vi "SV_Correction.vi"(8 "error in (no error)":errorcluster, 11 "Input Cluster":T3) -> (0 "error IO":errorcluster, 2 "Points for Array Overlay Out":T1(array[cluster]), 3 "Measurement Results":dbl[](array[numeric]))   [LabVIEW 2019, in "Algorithm.lvclass"]
uses:
  FrameworkOverrides/Algorithm.lvclass
  <vilib>/vision/NI_Vision_Development_Module.lvlib
  <vilib>/vision/Image Controls.llb/IMAQ Image.ctl
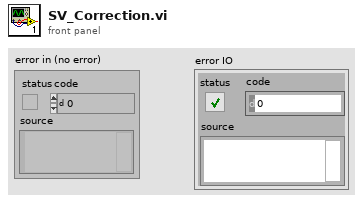
[diagram p1: front panel]
types:
  T1 = cluster{"Points for Arrow Overlay[0]":cluster{"X":sgl, "Y":sgl}, "Points for Arrow Overlay[1]":cluster{"X":sgl, "Y":sgl}, "Points for Arrow Overlay[2]":cluster{"X":sgl, "Y":sgl}, "Points for Arrow Overlay[3]":cluster{"X":sgl, "Y":sgl}}[]
  T2 = typedef "IMAQ Image.ctl" = refnum<image>
  T3 = cluster{"Side Calibration Image":T2, "Part Name":string, "Measurement Names Array":string[], "Measurement Results":dbl[], "Points for Array Overlay in":cluster{"Points for Arrow Overlay[0]":cluster{"X":sgl, "Y":sgl}, "Points for Arrow Overlay[1]":cluster{"X":sgl, "Y":sgl}, "Points for Arrow Overlay[2]":cluster{"X":sgl, "Y":sgl}, "Points for Arrow Overlay[3]":cluster{"X":sgl, "Y":sgl}}[]}
  T4 = cluster{"Points for Arrow Overlay[0]":cluster{"X":sgl, "Y":sgl}, "Points for Arrow Overlay[1]":cluster{"X":sgl, "Y":sgl}, "Points for Arrow Overlay[2]":cluster{"X":sgl, "Y":sgl}, "Points for Arrow Overlay[3]":cluster{"X":sgl, "Y":sgl}}
  T5 = cluster{"Pixel Coordinates":cluster{"X":sgl, "Y":sgl}, "Pixel Coordinates":cluster{"X":sgl, "Y":sgl}, "Points for Arrow Overlay[2]":cluster{"X":sgl, "Y":sgl}, "Points for Arrow Overlay[3]":cluster{"X":sgl, "Y":sgl}}
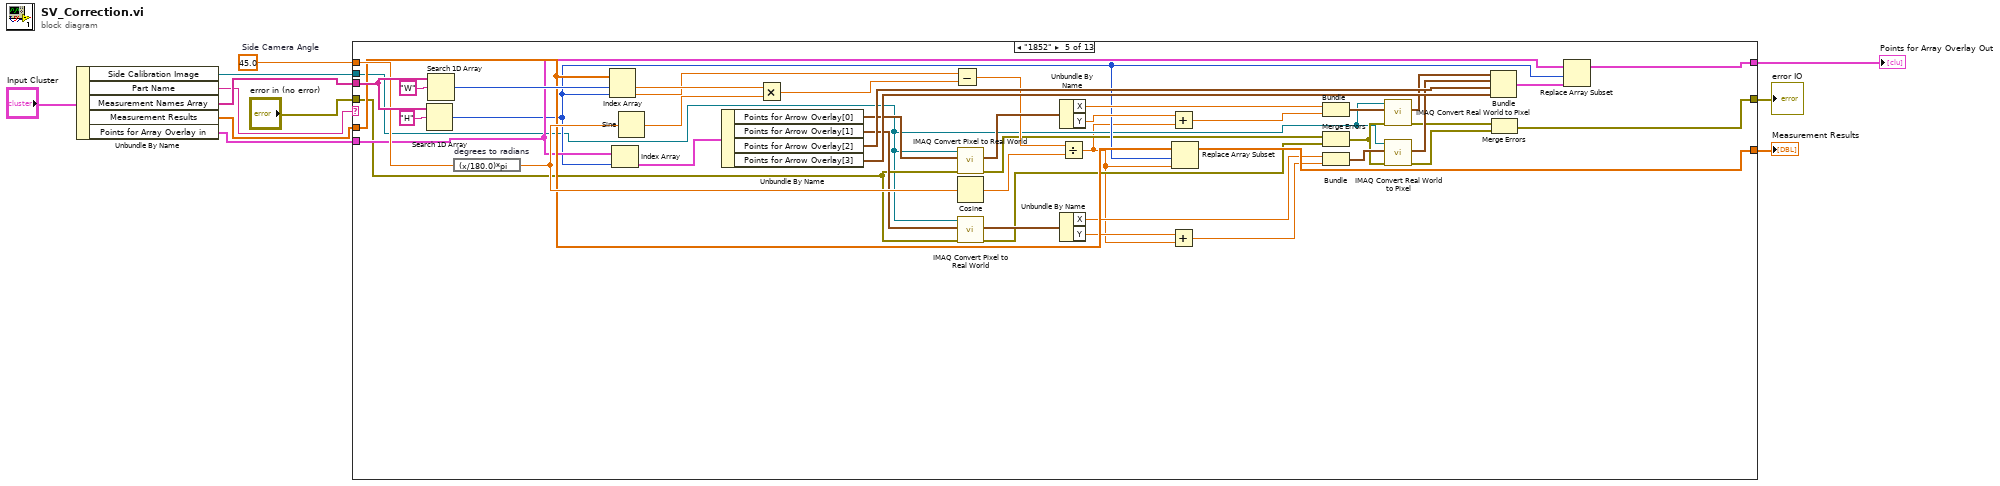
[diagram p0: block diagram]
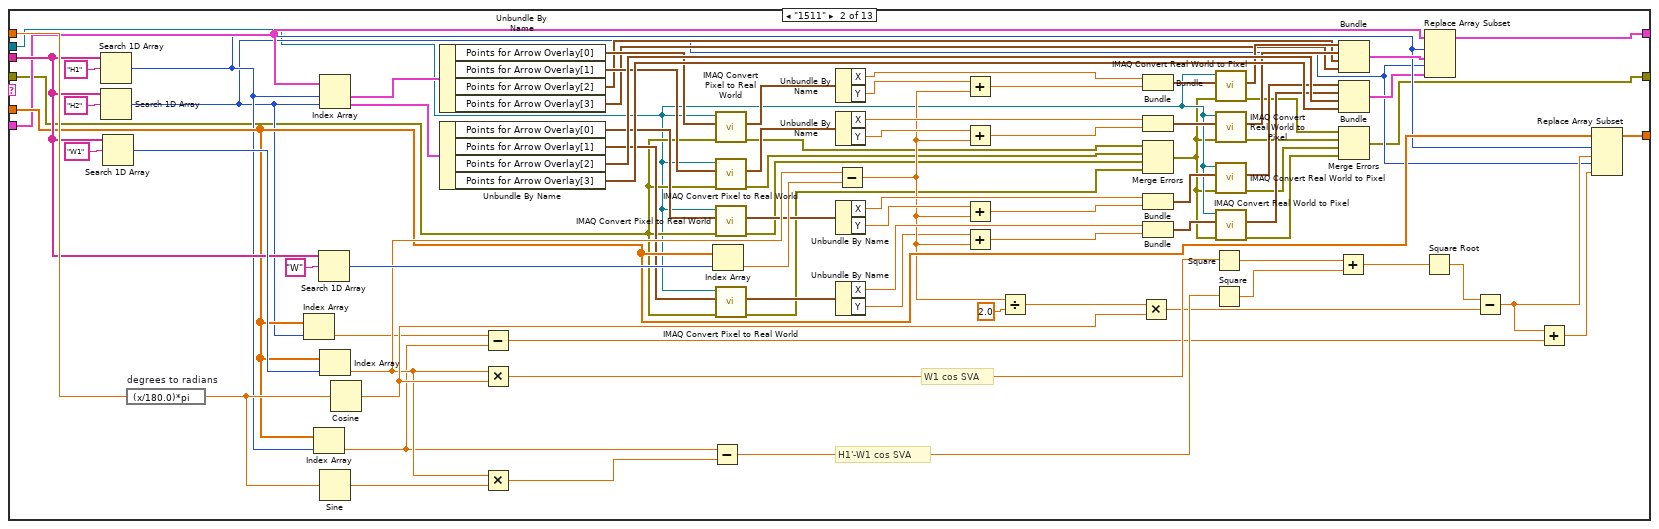
[diagram p3: hidden frame]
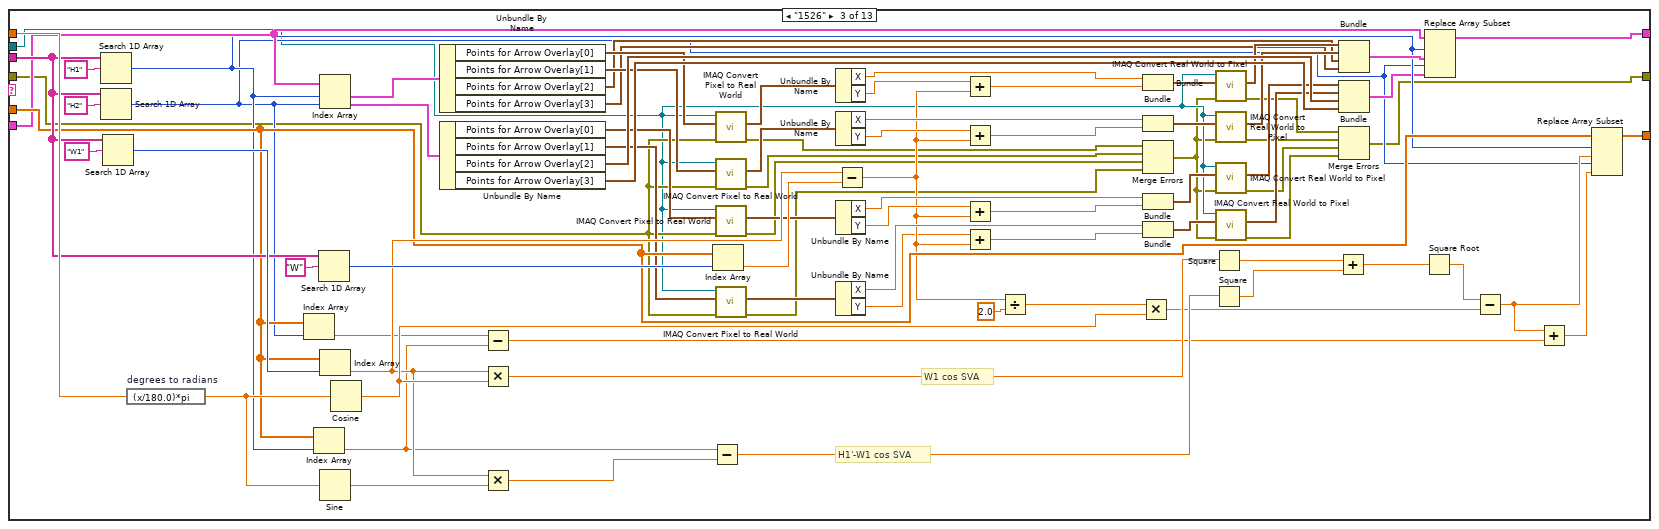
[diagram p4: hidden frame]
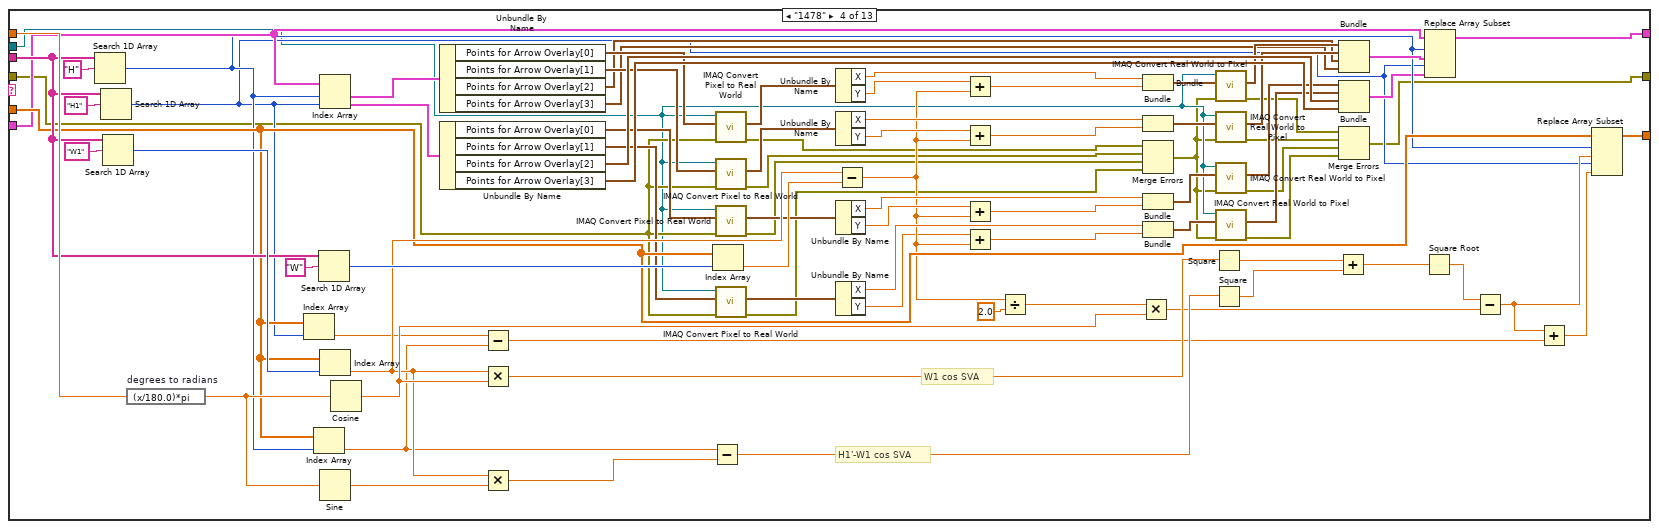
[diagram p5: hidden frame]
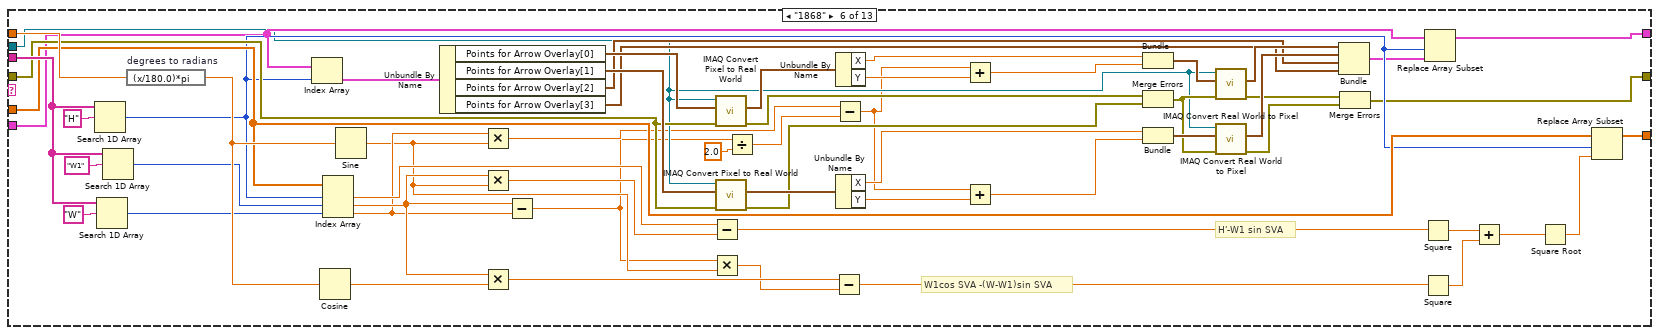
[diagram p6: hidden frame]
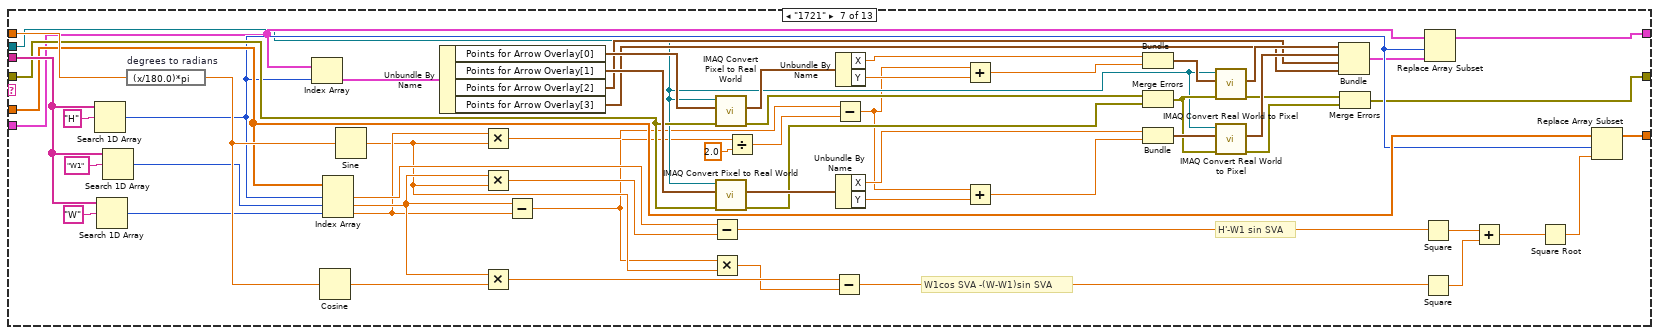
[diagram p7: hidden frame]
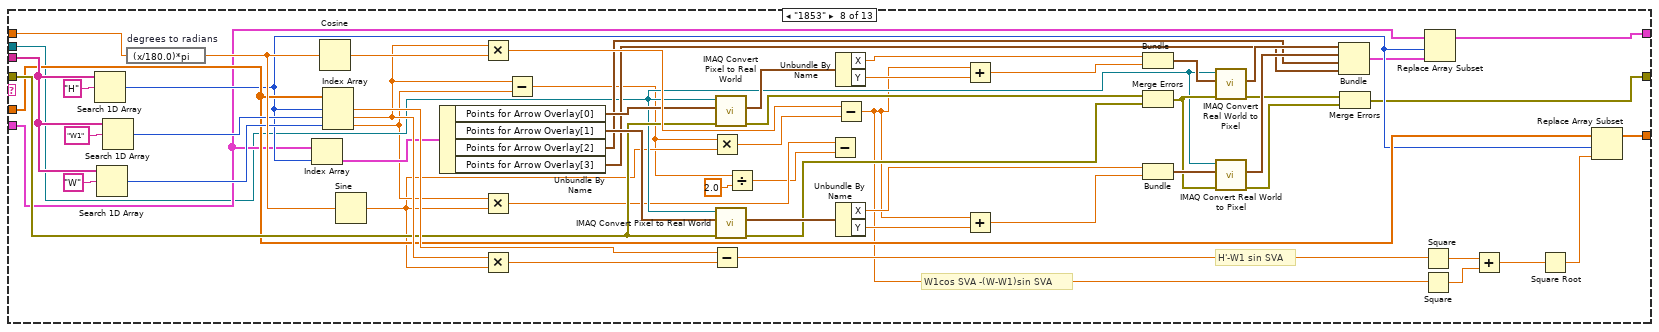
[diagram p8: hidden frame]
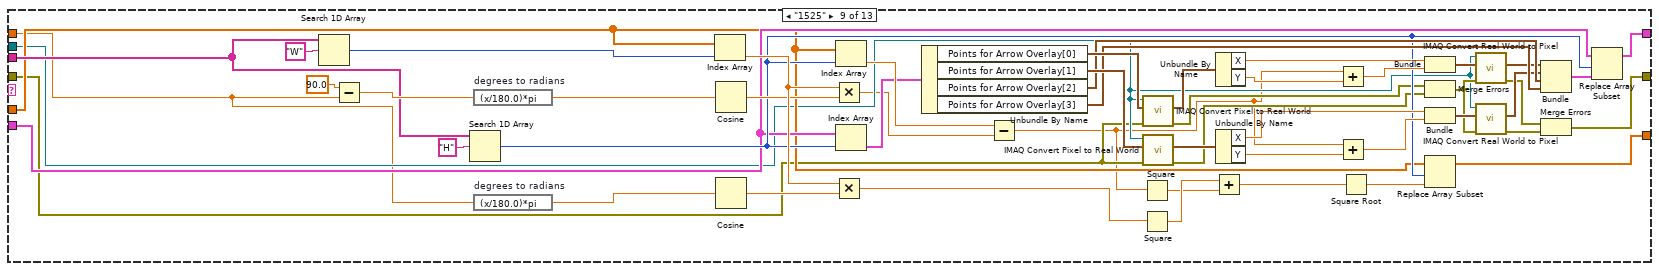
[diagram p9: hidden frame]
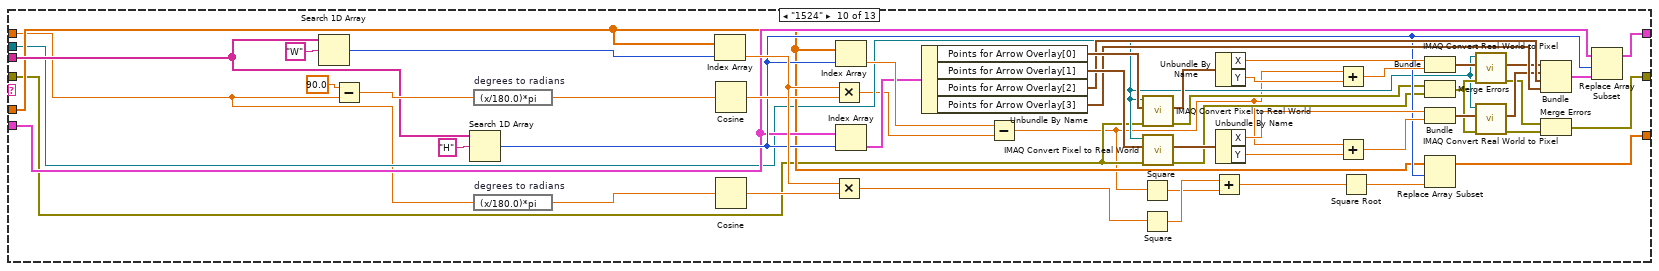
[diagram p10: hidden frame]
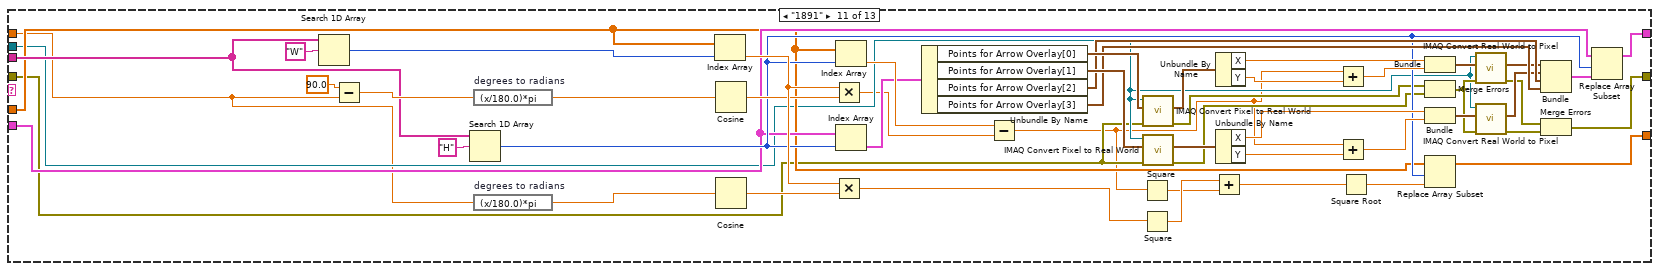
[diagram p11: hidden frame]
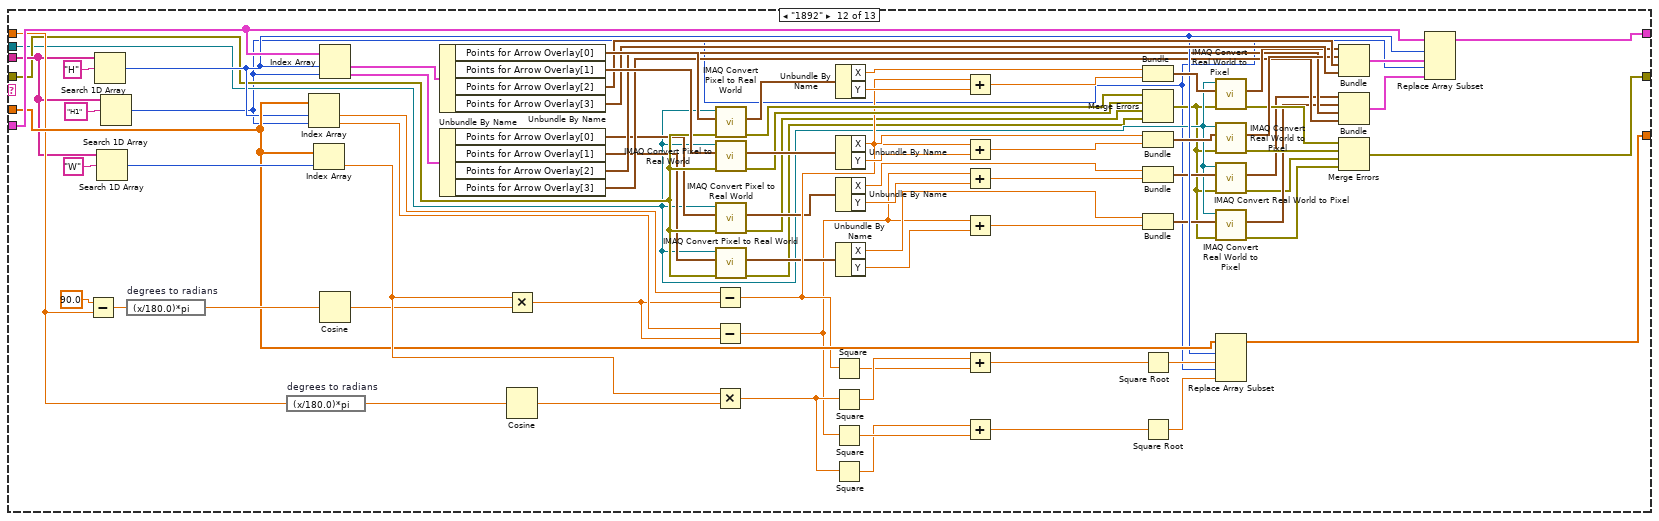
[diagram p12: hidden frame]
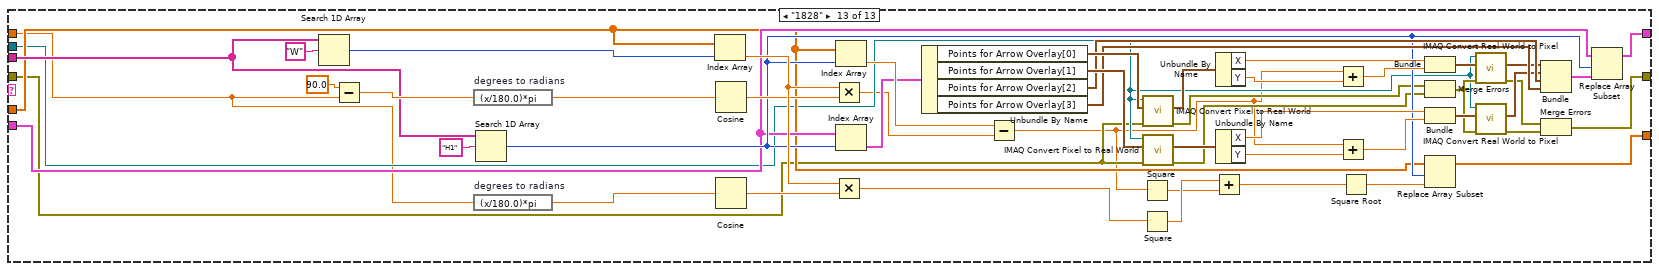
[diagram p13: hidden frame]
diagram:
  w10 = 45.0  # Side Camera Angle
  n1 = Unbundle By Name("Input Cluster") -> ("Side Calibration Image"=w5:T2, "Part Name"=w8:string, "Measurement Names Array"=w9:string[], "Measurement Results"=w7:dbl[], "Points for Array Overlay in"=w4:T1)
  n2 = case shown="\"1852\"" w8 {
    tunnel: w10 -> [_ w83 w166 w249 w299 w347 w405 w463 w487 w538 w589 w675 w721]
    tunnel: w9 -> [_ w78 w161 w244 w303 w355 w413 w471 w491 w542 w593 w669 w725]
    tunnel: w7 -> [w13 w71 w154 w237 w295 w325 w383 w441 w489 w540 w591 w676 w723]
    tunnel: [w13 w69 w152 w235 w294 w324 w382 w440 w485 w536 w587 w674 w719] -> w6
    tunnel: w5 -> [_ w20 w103 w186 w265 w316 w374 w432 w488 w539 w590 w643 w722]
    tunnel: w4 -> [w12 w34 w117 w200 w293 w322 w380 w438 w490 w541 w592 w677 w724]
    tunnel: [w12 w27 w110 w193 w273 w320 w378 w436 w484 w535 w586 w673 w718] -> w3
    tunnel: "error in (no error)" -> [w14 w26 w109 w192 w272 w334 w392 w450 w486 w537 w588 w657 w720]
    tunnel: [w14 w21 w104 w187 w266 w317 w375 w433 w483 w534 w585 w672 w717] -> w1
    frame "False", Default {
    }
    frame "1511" {
      # "H1'-W1 cos SVA"
      # "W1 cos SVA"
      n3 = Search 1D Array(1D array=w78, element="H1") -> (index of element=w32:i32)  [unwired: 1 in]
      n4 = Search 1D Array(1D array=w78, element="H2") -> (index of element=w28:i32)  [unwired: 1 in]
      n5 = Search 1D Array(1D array=w78, element="W1") -> (index of element=w80:i32)  [unwired: 1 in]
      n6 = expression code="(x/180.0)*pi" "degrees to radians"(w83) -> (w97:dbl)
      n7 = Index Array(array=w71, index=w28) -> (element=w72:dbl)
      n8 = Index Array(array=w71, index=w32) -> (element=w73:dbl)
      n9 = Search 1D Array(1D array=w78, element="W") -> (index of element=w79:i32)  [unwired: 1 in]
      n10 = Index Array(array=w34, index #1=w32, index #2=w28) -> (element #1=w67:T4, element #2=w66:T4)
      n11 = Index Array(array=w71, index=w80) -> (element=w75:dbl)
      n12 = Sine(x=w97) -> (sin(x)=w95:dbl)
      n13 = Cosine(x=w97) -> (cos(x)=w87:dbl)
      n14 = Unbundle By Name(w67) -> ("Points for Arrow Overlay[0]"=w63:cluster{"X":sgl, "Y":sgl}, "Points for Arrow Overlay[1]"=w62:cluster{"X":sgl, "Y":sgl}, "Points for Arrow Overlay[2]"=w49:cluster{"X":sgl, "Y":sgl}, "Points for Arrow Overlay[3]"=w48:cluster{"X":sgl, "Y":sgl})
      n15 = Unbundle By Name(w66) -> ("Points for Arrow Overlay[0]"=w47:cluster{"X":sgl, "Y":sgl}, "Points for Arrow Overlay[1]"=w46:cluster{"X":sgl, "Y":sgl}, "Points for Arrow Overlay[2]"=w64:cluster{"X":sgl, "Y":sgl}, "Points for Arrow Overlay[3]"=w65:cluster{"X":sgl, "Y":sgl})
      n16 = Subtract(x=w72, y=w73) -> (x-y=w84:dbl)
      n17 = Multiply(x=w75, y=w87) -> (x*y=w96:dbl)
      n18 = Multiply(x=w75, y=w95) -> (x*y=w94:dbl)
      n19 = Subtract(x=w73, y=w94) -> (x-y=w93:dbl)
      n20 = Index Array(array=w71, index=w79) -> (element=w74:dbl)
      n21 = call "IMAQ Convert Pixel to Real World"("error in (no error)"=w26, "Pixel Coordinates"=w63, "Calibrated Image"=w20) -> ("error out"=w19:errorcluster, "Real World Coordinates"=w61:cluster{"X":sgl, "Y":sgl})  [unwired: 3 in, 4 out]
      n22 = call "IMAQ Convert Pixel to Real World"("error in (no error)"=w26, "Pixel Coordinates"=w62, "Calibrated Image"=w20) -> ("error out"=w18:errorcluster, "Real World Coordinates"=w56:cluster{"X":sgl, "Y":sgl})  [unwired: 3 in, 4 out]
      n23 = call "IMAQ Convert Pixel to Real World"("error in (no error)"=w26, "Pixel Coordinates"=w47, "Calibrated Image"=w20) -> ("error out"=w17:errorcluster, "Real World Coordinates"=w45:cluster{"X":sgl, "Y":sgl})  [unwired: 3 in, 4 out]
      n24 = call "IMAQ Convert Pixel to Real World"("error in (no error)"=w26, "Pixel Coordinates"=w46, "Calibrated Image"=w20) -> ("error out"=w16:errorcluster, "Real World Coordinates"=w44:cluster{"X":sgl, "Y":sgl})  [unwired: 3 in, 4 out]
      n25 = Unbundle By Name(w61) -> ("X"=w60:sgl, "Y"=w59:sgl)
      n26 = Unbundle By Name(w56) -> ("X"=w55:sgl, "Y"=w54:sgl)
      n27 = Unbundle By Name(w45) -> ("X"=w43:sgl, "Y"=w42:sgl)
      n28 = Unbundle By Name(w44) -> ("X"=w41:sgl, "Y"=w38:sgl)
      n29 = Subtract(x=w75, y=w74) -> (x-y=w39:dbl)
      n30 = Add(x=w59, y=w39) -> (x+y=w58:dbl)
      n31 = Add(x=w54, y=w39) -> (x+y=w57:dbl)
      n32 = Add(x=w42, y=w39) -> (x+y=w40:dbl)
      n33 = Add(x=w38, y=w39) -> (x+y=w37:dbl)
      n34 = Divide(x=w39, y=2.0) -> (x/y=w88:dbl)
      n35 = Multiply(x=w88, y=w87) -> (x*y=w85:dbl)
      n36 = Bundle("X"=w60, w58) -> (w53:cluster{"X":sgl, dbl})  [unwired: 1 in]
      n37 = Bundle("X"=w55, w57) -> (w52:cluster{"X":sgl, dbl})  [unwired: 1 in]
      n38 = Merge Errors(w19, w18, w17, w16) -> (w15:errorcluster)
      n39 = Bundle("X"=w43, w40) -> (w36:cluster{"X":sgl, dbl})  [unwired: 1 in]
      n40 = Bundle("X"=w41, w37) -> (w35:cluster{"X":sgl, dbl})  [unwired: 1 in]
      n41 = Square(x=w96) -> (x^2=w92:dbl)
      n42 = Square(x=w93) -> (x^2=w91:dbl)
      n43 = call "IMAQ Convert Real World to Pixel"("error in (no error)"=w15, "Real World Coordinates"=w53, "Calibrated Image"=w20) -> ("error out"=w25:errorcluster, "Pixel Coordinates"=w51:cluster{"X":sgl, "Y":sgl})  [unwired: 3 in, 4 out]
      n44 = call "IMAQ Convert Real World to Pixel"("error in (no error)"=w15, "Real World Coordinates"=w52, "Calibrated Image"=w20) -> ("error out"=w24:errorcluster, "Pixel Coordinates"=w50:cluster{"X":sgl, "Y":sgl})  [unwired: 3 in, 4 out]
      n45 = call "IMAQ Convert Real World to Pixel"("error in (no error)"=w15, "Real World Coordinates"=w36, "Calibrated Image"=w20) -> ("error out"=w23:errorcluster, "Pixel Coordinates"=w31:cluster{"X":sgl, "Y":sgl})  [unwired: 3 in, 4 out]
      n46 = call "IMAQ Convert Real World to Pixel"("error in (no error)"=w15, "Real World Coordinates"=w35, "Calibrated Image"=w20) -> ("error out"=w22:errorcluster, "Pixel Coordinates"=w30:cluster{"X":sgl, "Y":sgl})  [unwired: 3 in, 4 out]
      n47 = Add(x=w92, y=w91) -> (x+y=w90:dbl)
      n48 = Bundle("Pixel Coordinates"=w51, "Pixel Coordinates"=w50, "Points for Arrow Overlay[2]"=w49, "Points for Arrow Overlay[3]"=w48) -> (w33:T5)  [unwired: 1 in]
      n49 = Bundle("Pixel Coordinates"=w31, "Pixel Coordinates"=w30, "Points for Arrow Overlay[2]"=w64, "Points for Arrow Overlay[3]"=w65) -> (w29:T5)  [unwired: 1 in]
      n50 = Merge Errors(w25, w24, w23, w22) -> (w21:errorcluster)
      n51 = Square Root(x=w90) -> (sqrt(x)=w86:dbl)
      n52 = Replace Array Subset(array=w34, new element #1=w33, index #1=w32, new element #2=w29, index #2=w28) -> (w27:T1)
      n53 = Subtract(x=w86, y=w85) -> (x-y=w70:dbl)
      n54 = Add(x=w70, y=w84) -> (x+y=w68:dbl)
      n55 = Replace Array Subset(array=w71, new element #1=w70, index #1=w32, new element #2=w68, index #2=w28) -> (w69:dbl[])
    }
    frame "1526" {
      # "H1'-W1 cos SVA"
      # "W1 cos SVA"
      n56 = Search 1D Array(1D array=w161, element="H1") -> (index of element=w115:i32)  [unwired: 1 in]
      n57 = Search 1D Array(1D array=w161, element="H2") -> (index of element=w111:i32)  [unwired: 1 in]
      n58 = Search 1D Array(1D array=w161, element="W1") -> (index of element=w163:i32)  [unwired: 1 in]
      n59 = expression code="(x/180.0)*pi" "degrees to radians"(w166) -> (w180:dbl)
      n60 = Index Array(array=w154, index=w111) -> (element=w155:dbl)
      n61 = Index Array(array=w154, index=w115) -> (element=w156:dbl)
      n62 = Search 1D Array(1D array=w161, element="W") -> (index of element=w162:i32)  [unwired: 1 in]
      n63 = Index Array(array=w117, index #1=w115, index #2=w111) -> (element #1=w150:T4, element #2=w149:T4)
      n64 = Index Array(array=w154, index=w163) -> (element=w158:dbl)
      n65 = Sine(x=w180) -> (sin(x)=w178:dbl)
      n66 = Cosine(x=w180) -> (cos(x)=w170:dbl)
      n67 = Unbundle By Name(w150) -> ("Points for Arrow Overlay[0]"=w146:cluster{"X":sgl, "Y":sgl}, "Points for Arrow Overlay[1]"=w145:cluster{"X":sgl, "Y":sgl}, "Points for Arrow Overlay[2]"=w132:cluster{"X":sgl, "Y":sgl}, "Points for Arrow Overlay[3]"=w131:cluster{"X":sgl, "Y":sgl})
      n68 = Unbundle By Name(w149) -> ("Points for Arrow Overlay[0]"=w130:cluster{"X":sgl, "Y":sgl}, "Points for Arrow Overlay[1]"=w129:cluster{"X":sgl, "Y":sgl}, "Points for Arrow Overlay[2]"=w147:cluster{"X":sgl, "Y":sgl}, "Points for Arrow Overlay[3]"=w148:cluster{"X":sgl, "Y":sgl})
      n69 = Subtract(x=w155, y=w156) -> (x-y=w167:dbl)
      n70 = Multiply(x=w158, y=w170) -> (x*y=w179:dbl)
      n71 = Multiply(x=w158, y=w178) -> (x*y=w177:dbl)
      n72 = Subtract(x=w156, y=w177) -> (x-y=w176:dbl)
      n73 = Index Array(array=w154, index=w162) -> (element=w157:dbl)
      n74 = call "IMAQ Convert Pixel to Real World"("error in (no error)"=w109, "Pixel Coordinates"=w146, "Calibrated Image"=w103) -> ("error out"=w102:errorcluster, "Real World Coordinates"=w144:cluster{"X":sgl, "Y":sgl})  [unwired: 3 in, 4 out]
      n75 = call "IMAQ Convert Pixel to Real World"("error in (no error)"=w109, "Pixel Coordinates"=w145, "Calibrated Image"=w103) -> ("error out"=w101:errorcluster, "Real World Coordinates"=w139:cluster{"X":sgl, "Y":sgl})  [unwired: 3 in, 4 out]
      n76 = call "IMAQ Convert Pixel to Real World"("error in (no error)"=w109, "Pixel Coordinates"=w130, "Calibrated Image"=w103) -> ("error out"=w100:errorcluster, "Real World Coordinates"=w128:cluster{"X":sgl, "Y":sgl})  [unwired: 3 in, 4 out]
      n77 = call "IMAQ Convert Pixel to Real World"("error in (no error)"=w109, "Pixel Coordinates"=w129, "Calibrated Image"=w103) -> ("error out"=w99:errorcluster, "Real World Coordinates"=w127:cluster{"X":sgl, "Y":sgl})  [unwired: 3 in, 4 out]
      n78 = Unbundle By Name(w144) -> ("X"=w143:sgl, "Y"=w142:sgl)
      n79 = Unbundle By Name(w139) -> ("X"=w138:sgl, "Y"=w137:sgl)
      n80 = Unbundle By Name(w128) -> ("X"=w126:sgl, "Y"=w125:sgl)
      n81 = Unbundle By Name(w127) -> ("X"=w124:sgl, "Y"=w121:sgl)
      n82 = Subtract(x=w158, y=w157) -> (x-y=w122:dbl)
      n83 = Add(x=w142, y=w122) -> (x+y=w141:dbl)
      n84 = Add(x=w137, y=w122) -> (x+y=w140:dbl)
      n85 = Add(x=w125, y=w122) -> (x+y=w123:dbl)
      n86 = Add(x=w121, y=w122) -> (x+y=w120:dbl)
      n87 = Divide(x=w122, y=2.0) -> (x/y=w171:dbl)
      n88 = Multiply(x=w171, y=w170) -> (x*y=w168:dbl)
      n89 = Bundle("X"=w143, w141) -> (w136:cluster{"X":sgl, dbl})  [unwired: 1 in]
      n90 = Bundle("X"=w138, w140) -> (w135:cluster{"X":sgl, dbl})  [unwired: 1 in]
      n91 = Merge Errors(w102, w101, w100, w99) -> (w98:errorcluster)
      n92 = Bundle("X"=w126, w123) -> (w119:cluster{"X":sgl, dbl})  [unwired: 1 in]
      n93 = Bundle("X"=w124, w120) -> (w118:cluster{"X":sgl, dbl})  [unwired: 1 in]
      n94 = Square(x=w179) -> (x^2=w175:dbl)
      n95 = Square(x=w176) -> (x^2=w174:dbl)
      n96 = call "IMAQ Convert Real World to Pixel"("error in (no error)"=w98, "Real World Coordinates"=w136, "Calibrated Image"=w103) -> ("error out"=w108:errorcluster, "Pixel Coordinates"=w134:cluster{"X":sgl, "Y":sgl})  [unwired: 3 in, 4 out]
      n97 = call "IMAQ Convert Real World to Pixel"("error in (no error)"=w98, "Real World Coordinates"=w135, "Calibrated Image"=w103) -> ("error out"=w107:errorcluster, "Pixel Coordinates"=w133:cluster{"X":sgl, "Y":sgl})  [unwired: 3 in, 4 out]
      n98 = call "IMAQ Convert Real World to Pixel"("error in (no error)"=w98, "Real World Coordinates"=w119, "Calibrated Image"=w103) -> ("error out"=w106:errorcluster, "Pixel Coordinates"=w114:cluster{"X":sgl, "Y":sgl})  [unwired: 3 in, 4 out]
      n99 = call "IMAQ Convert Real World to Pixel"("error in (no error)"=w98, "Real World Coordinates"=w118, "Calibrated Image"=w103) -> ("error out"=w105:errorcluster, "Pixel Coordinates"=w113:cluster{"X":sgl, "Y":sgl})  [unwired: 3 in, 4 out]
      n100 = Add(x=w175, y=w174) -> (x+y=w173:dbl)
      n101 = Bundle("Pixel Coordinates"=w134, "Pixel Coordinates"=w133, "Points for Arrow Overlay[2]"=w132, "Points for Arrow Overlay[3]"=w131) -> (w116:T5)  [unwired: 1 in]
      n102 = Bundle("Pixel Coordinates"=w114, "Pixel Coordinates"=w113, "Points for Arrow Overlay[2]"=w147, "Points for Arrow Overlay[3]"=w148) -> (w112:T5)  [unwired: 1 in]
      n103 = Merge Errors(w108, w107, w106, w105) -> (w104:errorcluster)
      n104 = Square Root(x=w173) -> (sqrt(x)=w169:dbl)
      n105 = Replace Array Subset(array=w117, new element #1=w116, index #1=w115, new element #2=w112, index #2=w111) -> (w110:T1)
      n106 = Subtract(x=w169, y=w168) -> (x-y=w153:dbl)
      n107 = Add(x=w153, y=w167) -> (x+y=w151:dbl)
      n108 = Replace Array Subset(array=w154, new element #1=w153, index #1=w115, new element #2=w151, index #2=w111) -> (w152:dbl[])
    }
    frame "1478" {
      # "H1'-W1 cos SVA"
      # "W1 cos SVA"
      n109 = Search 1D Array(1D array=w244, element="H") -> (index of element=w198:i32)  [unwired: 1 in]
      n110 = Search 1D Array(1D array=w244, element="H1") -> (index of element=w194:i32)  [unwired: 1 in]
      n111 = Search 1D Array(1D array=w244, element="W1") -> (index of element=w246:i32)  [unwired: 1 in]
      n112 = expression code="(x/180.0)*pi" "degrees to radians"(w249) -> (w263:dbl)
      n113 = Index Array(array=w237, index=w194) -> (element=w238:dbl)
      n114 = Index Array(array=w237, index=w198) -> (element=w239:dbl)
      n115 = Search 1D Array(1D array=w244, element="W") -> (index of element=w245:i32)  [unwired: 1 in]
      n116 = Index Array(array=w200, index #1=w198, index #2=w194) -> (element #1=w233:T4, element #2=w232:T4)
      n117 = Index Array(array=w237, index=w246) -> (element=w241:dbl)
      n118 = Sine(x=w263) -> (sin(x)=w261:dbl)
      n119 = Cosine(x=w263) -> (cos(x)=w253:dbl)
      n120 = Unbundle By Name(w233) -> ("Points for Arrow Overlay[0]"=w229:cluster{"X":sgl, "Y":sgl}, "Points for Arrow Overlay[1]"=w228:cluster{"X":sgl, "Y":sgl}, "Points for Arrow Overlay[2]"=w215:cluster{"X":sgl, "Y":sgl}, "Points for Arrow Overlay[3]"=w214:cluster{"X":sgl, "Y":sgl})
      n121 = Unbundle By Name(w232) -> ("Points for Arrow Overlay[0]"=w213:cluster{"X":sgl, "Y":sgl}, "Points for Arrow Overlay[1]"=w212:cluster{"X":sgl, "Y":sgl}, "Points for Arrow Overlay[2]"=w230:cluster{"X":sgl, "Y":sgl}, "Points for Arrow Overlay[3]"=w231:cluster{"X":sgl, "Y":sgl})
      n122 = Subtract(x=w238, y=w239) -> (x-y=w250:dbl)
      n123 = Multiply(x=w241, y=w253) -> (x*y=w262:dbl)
      n124 = Multiply(x=w241, y=w261) -> (x*y=w260:dbl)
      n125 = Subtract(x=w239, y=w260) -> (x-y=w259:dbl)
      n126 = Index Array(array=w237, index=w245) -> (element=w240:dbl)
      n127 = call "IMAQ Convert Pixel to Real World"("error in (no error)"=w192, "Pixel Coordinates"=w229, "Calibrated Image"=w186) -> ("error out"=w185:errorcluster, "Real World Coordinates"=w227:cluster{"X":sgl, "Y":sgl})  [unwired: 3 in, 4 out]
      n128 = call "IMAQ Convert Pixel to Real World"("error in (no error)"=w192, "Pixel Coordinates"=w228, "Calibrated Image"=w186) -> ("error out"=w184:errorcluster, "Real World Coordinates"=w222:cluster{"X":sgl, "Y":sgl})  [unwired: 3 in, 4 out]
      n129 = call "IMAQ Convert Pixel to Real World"("error in (no error)"=w192, "Pixel Coordinates"=w213, "Calibrated Image"=w186) -> ("error out"=w183:errorcluster, "Real World Coordinates"=w211:cluster{"X":sgl, "Y":sgl})  [unwired: 3 in, 4 out]
      n130 = call "IMAQ Convert Pixel to Real World"("error in (no error)"=w192, "Pixel Coordinates"=w212, "Calibrated Image"=w186) -> ("error out"=w182:errorcluster, "Real World Coordinates"=w210:cluster{"X":sgl, "Y":sgl})  [unwired: 3 in, 4 out]
      n131 = Unbundle By Name(w227) -> ("X"=w226:sgl, "Y"=w225:sgl)
      n132 = Unbundle By Name(w222) -> ("X"=w221:sgl, "Y"=w220:sgl)
      n133 = Unbundle By Name(w211) -> ("X"=w209:sgl, "Y"=w208:sgl)
      n134 = Unbundle By Name(w210) -> ("X"=w207:sgl, "Y"=w204:sgl)
      n135 = Subtract(x=w241, y=w240) -> (x-y=w205:dbl)
      n136 = Add(x=w225, y=w205) -> (x+y=w224:dbl)
      n137 = Add(x=w220, y=w205) -> (x+y=w223:dbl)
      n138 = Add(x=w208, y=w205) -> (x+y=w206:dbl)
      n139 = Add(x=w204, y=w205) -> (x+y=w203:dbl)
      n140 = Divide(x=w205, y=2.0) -> (x/y=w254:dbl)
      n141 = Multiply(x=w254, y=w253) -> (x*y=w251:dbl)
      n142 = Bundle("X"=w226, w224) -> (w219:cluster{"X":sgl, dbl})  [unwired: 1 in]
      n143 = Bundle("X"=w221, w223) -> (w218:cluster{"X":sgl, dbl})  [unwired: 1 in]
      n144 = Merge Errors(w185, w184, w183, w182) -> (w181:errorcluster)
      n145 = Bundle("X"=w209, w206) -> (w202:cluster{"X":sgl, dbl})  [unwired: 1 in]
      n146 = Bundle("X"=w207, w203) -> (w201:cluster{"X":sgl, dbl})  [unwired: 1 in]
      n147 = Square(x=w262) -> (x^2=w258:dbl)
      n148 = Square(x=w259) -> (x^2=w257:dbl)
      n149 = call "IMAQ Convert Real World to Pixel"("error in (no error)"=w181, "Real World Coordinates"=w219, "Calibrated Image"=w186) -> ("error out"=w191:errorcluster, "Pixel Coordinates"=w217:cluster{"X":sgl, "Y":sgl})  [unwired: 3 in, 4 out]
      n150 = call "IMAQ Convert Real World to Pixel"("error in (no error)"=w181, "Real World Coordinates"=w218, "Calibrated Image"=w186) -> ("error out"=w190:errorcluster, "Pixel Coordinates"=w216:cluster{"X":sgl, "Y":sgl})  [unwired: 3 in, 4 out]
      n151 = call "IMAQ Convert Real World to Pixel"("error in (no error)"=w181, "Real World Coordinates"=w202, "Calibrated Image"=w186) -> ("error out"=w189:errorcluster, "Pixel Coordinates"=w197:cluster{"X":sgl, "Y":sgl})  [unwired: 3 in, 4 out]
      n152 = call "IMAQ Convert Real World to Pixel"("error in (no error)"=w181, "Real World Coordinates"=w201, "Calibrated Image"=w186) -> ("error out"=w188:errorcluster, "Pixel Coordinates"=w196:cluster{"X":sgl, "Y":sgl})  [unwired: 3 in, 4 out]
      n153 = Add(x=w258, y=w257) -> (x+y=w256:dbl)
      n154 = Bundle("Pixel Coordinates"=w217, "Pixel Coordinates"=w216, "Points for Arrow Overlay[2]"=w215, "Points for Arrow Overlay[3]"=w214) -> (w199:T5)  [unwired: 1 in]
      n155 = Bundle("Pixel Coordinates"=w197, "Pixel Coordinates"=w196, "Points for Arrow Overlay[2]"=w230, "Points for Arrow Overlay[3]"=w231) -> (w195:T5)  [unwired: 1 in]
      n156 = Merge Errors(w191, w190, w189, w188) -> (w187:errorcluster)
      n157 = Square Root(x=w256) -> (sqrt(x)=w252:dbl)
      n158 = Replace Array Subset(array=w200, new element #1=w199, index #1=w198, new element #2=w195, index #2=w194) -> (w193:T1)
      n159 = Subtract(x=w252, y=w251) -> (x-y=w236:dbl)
      n160 = Add(x=w236, y=w250) -> (x+y=w234:dbl)
      n161 = Replace Array Subset(array=w237, new element #1=w236, index #1=w198, new element #2=w234, index #2=w194) -> (w235:dbl[])
    }
    frame "1852" {
      n162 = Search 1D Array(1D array=w303, element="H") -> (index of element=w275:i32)  [unwired: 1 in]
      n163 = Search 1D Array(1D array=w303, element="W") -> (index of element=w300:i32)  [unwired: 1 in]
      n164 = expression code="(x/180.0)*pi" "degrees to radians"(w299) -> (w307:dbl)
      n165 = Index Array(array=w295, index #1=w300, index #2=w275) -> (element #1=w298:dbl, element #2=w297:dbl)
      n166 = Index Array(array=w293, index=w275) -> (element=w296:T4)
      n167 = Sine(x=w307) -> (sin(x)=w306:dbl)
      n168 = Unbundle By Name(w296) -> ("Points for Arrow Overlay[0]"=w290:cluster{"X":sgl, "Y":sgl}, "Points for Arrow Overlay[1]"=w289:cluster{"X":sgl, "Y":sgl}, "Points for Arrow Overlay[2]"=w291:cluster{"X":sgl, "Y":sgl}, "Points for Arrow Overlay[3]"=w292:cluster{"X":sgl, "Y":sgl})
      n169 = Multiply(x=w298, y=w306) -> (x*y=w305:dbl)
      n170 = Subtract(x=w297, y=w305) -> (x-y=w280:dbl)
      n171 = call "IMAQ Convert Pixel to Real World"("error in (no error)"=w272, "Pixel Coordinates"=w290, "Calibrated Image"=w265) -> ("error out"=w271:errorcluster, "Real World Coordinates"=w288:cluster{"X":sgl, "Y":sgl})  [unwired: 3 in, 4 out]
      n172 = Cosine(x=w307) -> (cos(x)=w304:dbl)
      n173 = call "IMAQ Convert Pixel to Real World"("error in (no error)"=w272, "Pixel Coordinates"=w289, "Calibrated Image"=w265) -> ("error out"=w270:errorcluster, "Real World Coordinates"=w287:cluster{"X":sgl, "Y":sgl})  [unwired: 3 in, 4 out]
      n174 = Unbundle By Name(w288) -> ("X"=w286:sgl, "Y"=w283:sgl)
      n175 = Divide(x=w280, y=w304) -> (x/y=w264:dbl)
      n176 = Unbundle By Name(w287) -> ("X"=w285:sgl, "Y"=w281:sgl)
      n177 = Add(x=w283, y=w264) -> (x+y=w284:dbl)
      n178 = Add(x=w281, y=w264) -> (x+y=w282:dbl)
      n179 = Replace Array Subset(array=w295, new element=w264, index=w275) -> (w294:dbl[])
      n180 = Bundle("X"=w286, w284) -> (w279:cluster{"X":sgl, dbl})  [unwired: 1 in]
      n181 = Merge Errors(w271, w270) -> (w267:errorcluster)
      n182 = Bundle("X"=w285, w282) -> (w278:cluster{"X":sgl, dbl})  [unwired: 1 in]
      n183 = call "IMAQ Convert Real World to Pixel"("error in (no error)"=w267, "Real World Coordinates"=w279, "Calibrated Image"=w265) -> ("error out"=w269:errorcluster, "Pixel Coordinates"=w277:cluster{"X":sgl, "Y":sgl})  [unwired: 3 in, 4 out]
      n184 = call "IMAQ Convert Real World to Pixel"("error in (no error)"=w267, "Real World Coordinates"=w278, "Calibrated Image"=w265) -> ("error out"=w268:errorcluster, "Pixel Coordinates"=w276:cluster{"X":sgl, "Y":sgl})  [unwired: 3 in, 4 out]
      n185 = Bundle("Pixel Coordinates"=w277, "Pixel Coordinates"=w276, "Points for Arrow Overlay[2]"=w291, "Points for Arrow Overlay[3]"=w292) -> (w274:T5)  [unwired: 1 in]
      n186 = Merge Errors(w269, w268) -> (w266:errorcluster)
      n187 = Replace Array Subset(array=w293, new element=w274, index=w275) -> (w273:T1)
    }
    frame "1868" {
      # "W1cos SVA -(W-W1)sin SVA"
      # "H'-W1 sin SVA"
      n188 = Search 1D Array(1D array=w355, element="H") -> (index of element=w323:i32)  [unwired: 1 in]
      n189 = Search 1D Array(1D array=w355, element="W") -> (index of element=w351:i32)  [unwired: 1 in]
      n190 = Search 1D Array(1D array=w355, element="W1") -> (index of element=w352:i32)  [unwired: 1 in]
      n191 = expression code="(x/180.0)*pi" "degrees to radians"(w347) -> (w365:dbl)
      n192 = Index Array(array=w322, index=w323) -> (element=w348:T4)
      n193 = Cosine(x=w365) -> (cos(x)=w364:dbl)
      n194 = Index Array(array=w325, index #1=w323, index #2=w352, index #3=w351) -> (element #1=w350:dbl, element #2=w349:dbl, element #3=w315:dbl)
      n195 = Sine(x=w365) -> (sin(x)=w314:dbl)
      n196 = Unbundle By Name(w348) -> ("Points for Arrow Overlay[0]"=w346:cluster{"X":sgl, "Y":sgl}, "Points for Arrow Overlay[1]"=w345:cluster{"X":sgl, "Y":sgl}, "Points for Arrow Overlay[2]"=w328:cluster{"X":sgl, "Y":sgl}, "Points for Arrow Overlay[3]"=w327:cluster{"X":sgl, "Y":sgl})
      n197 = Multiply(x=w315, y=w314) -> (x*y=w312:dbl)
      n198 = Multiply(x=w349, y=w314) -> (x*y=w313:dbl)
      n199 = Multiply(x=w349, y=w364) -> (x*y=w363:dbl)
      n200 = Subtract(x=w349, y=w315) -> (x-y=w310:dbl)
      n201 = Subtract(x=w350, y=w313) -> (x-y=w358:dbl)
      n202 = Multiply(x=w310, y=w314) -> (x*y=w357:dbl)
      n203 = call "IMAQ Convert Pixel to Real World"("error in (no error)"=w334, "Pixel Coordinates"=w346, "Calibrated Image"=w316) -> ("error out"=w333:errorcluster, "Real World Coordinates"=w344:cluster{"X":sgl, "Y":sgl})  [unwired: 3 in, 4 out]
      n204 = call "IMAQ Convert Pixel to Real World"("error in (no error)"=w334, "Pixel Coordinates"=w345, "Calibrated Image"=w316) -> ("error out"=w332:errorcluster, "Real World Coordinates"=w343:cluster{"X":sgl, "Y":sgl})  [unwired: 3 in, 4 out]
      n205 = Divide(x=w310, y=2.0) -> (x/y=w308:dbl)
      n206 = Subtract(x=w363, y=w357) -> (x-y=w362:dbl)
      n207 = Subtract(x=w312, y=w308) -> (x-y=w311:dbl)
      n208 = Unbundle By Name(w344) -> ("X"=w342:sgl, "Y"=w341:sgl)
      n209 = Unbundle By Name(w343) -> ("X"=w337:sgl, "Y"=w339:sgl)
      n210 = Add(x=w311, y=w341) -> (x+y=w340:dbl)
      n211 = Add(x=w311, y=w339) -> (x+y=w338:dbl)
      n212 = Bundle("X"=w342, w340) -> (w336:cluster{"X":sgl, dbl})  [unwired: 1 in]
      n213 = Merge Errors(w333, w332) -> (w331:errorcluster)
      n214 = Bundle("X"=w337, w338) -> (w335:cluster{"X":sgl, dbl})  [unwired: 1 in]
      n215 = call "IMAQ Convert Real World to Pixel"("error in (no error)"=w331, "Real World Coordinates"=w336, "Calibrated Image"=w316) -> ("error out"=w319:errorcluster, "Pixel Coordinates"=w330:cluster{"X":sgl, "Y":sgl})  [unwired: 3 in, 4 out]
      n216 = call "IMAQ Convert Real World to Pixel"("error in (no error)"=w331, "Real World Coordinates"=w335, "Calibrated Image"=w316) -> ("error out"=w318:errorcluster, "Pixel Coordinates"=w329:cluster{"X":sgl, "Y":sgl})  [unwired: 3 in, 4 out]
      n217 = Bundle("Pixel Coordinates"=w330, "Pixel Coordinates"=w329, "Points for Arrow Overlay[2]"=w328, "Points for Arrow Overlay[3]"=w327) -> (w321:T5)  [unwired: 1 in]
      n218 = Merge Errors(w319, w318) -> (w317:errorcluster)
      n219 = Square(x=w358) -> (x^2=w361:dbl)
      n220 = Square(x=w362) -> (x^2=w360:dbl)
      n221 = Replace Array Subset(array=w322, new element=w321, index=w323) -> (w320:T1)
      n222 = Add(x=w361, y=w360) -> (x+y=w359:dbl)
      n223 = Square Root(x=w359) -> (sqrt(x)=w326:dbl)
      n224 = Replace Array Subset(array=w325, new element=w326, index=w323) -> (w324:dbl[])
    }
    frame "1721" {
      # "W1cos SVA -(W-W1)sin SVA"
      # "H'-W1 sin SVA"
      n225 = Search 1D Array(1D array=w413, element="H") -> (index of element=w381:i32)  [unwired: 1 in]
      n226 = Search 1D Array(1D array=w413, element="W") -> (index of element=w409:i32)  [unwired: 1 in]
      n227 = Search 1D Array(1D array=w413, element="W1") -> (index of element=w410:i32)  [unwired: 1 in]
      n228 = expression code="(x/180.0)*pi" "degrees to radians"(w405) -> (w423:dbl)
      n229 = Index Array(array=w380, index=w381) -> (element=w406:T4)
      n230 = Cosine(x=w423) -> (cos(x)=w422:dbl)
      n231 = Index Array(array=w383, index #1=w381, index #2=w410, index #3=w409) -> (element #1=w408:dbl, element #2=w407:dbl, element #3=w373:dbl)
      n232 = Sine(x=w423) -> (sin(x)=w372:dbl)
      n233 = Unbundle By Name(w406) -> ("Points for Arrow Overlay[0]"=w404:cluster{"X":sgl, "Y":sgl}, "Points for Arrow Overlay[1]"=w403:cluster{"X":sgl, "Y":sgl}, "Points for Arrow Overlay[2]"=w386:cluster{"X":sgl, "Y":sgl}, "Points for Arrow Overlay[3]"=w385:cluster{"X":sgl, "Y":sgl})
      n234 = Multiply(x=w373, y=w372) -> (x*y=w370:dbl)
      n235 = Multiply(x=w407, y=w372) -> (x*y=w371:dbl)
      n236 = Multiply(x=w407, y=w422) -> (x*y=w421:dbl)
      n237 = Subtract(x=w407, y=w373) -> (x-y=w368:dbl)
      n238 = Subtract(x=w408, y=w371) -> (x-y=w416:dbl)
      n239 = Multiply(x=w368, y=w372) -> (x*y=w415:dbl)
      n240 = call "IMAQ Convert Pixel to Real World"("error in (no error)"=w392, "Pixel Coordinates"=w404, "Calibrated Image"=w374) -> ("error out"=w391:errorcluster, "Real World Coordinates"=w402:cluster{"X":sgl, "Y":sgl})  [unwired: 3 in, 4 out]
      n241 = call "IMAQ Convert Pixel to Real World"("error in (no error)"=w392, "Pixel Coordinates"=w403, "Calibrated Image"=w374) -> ("error out"=w390:errorcluster, "Real World Coordinates"=w401:cluster{"X":sgl, "Y":sgl})  [unwired: 3 in, 4 out]
      n242 = Divide(x=w368, y=2.0) -> (x/y=w366:dbl)
      n243 = Subtract(x=w421, y=w415) -> (x-y=w420:dbl)
      n244 = Subtract(x=w370, y=w366) -> (x-y=w369:dbl)
      n245 = Unbundle By Name(w402) -> ("X"=w400:sgl, "Y"=w399:sgl)
      n246 = Unbundle By Name(w401) -> ("X"=w395:sgl, "Y"=w397:sgl)
      n247 = Add(x=w369, y=w399) -> (x+y=w398:dbl)
      n248 = Add(x=w369, y=w397) -> (x+y=w396:dbl)
      n249 = Bundle("X"=w400, w398) -> (w394:cluster{"X":sgl, dbl})  [unwired: 1 in]
      n250 = Merge Errors(w391, w390) -> (w389:errorcluster)
      n251 = Bundle("X"=w395, w396) -> (w393:cluster{"X":sgl, dbl})  [unwired: 1 in]
      n252 = call "IMAQ Convert Real World to Pixel"("error in (no error)"=w389, "Real World Coordinates"=w394, "Calibrated Image"=w374) -> ("error out"=w377:errorcluster, "Pixel Coordinates"=w388:cluster{"X":sgl, "Y":sgl})  [unwired: 3 in, 4 out]
      n253 = call "IMAQ Convert Real World to Pixel"("error in (no error)"=w389, "Real World Coordinates"=w393, "Calibrated Image"=w374) -> ("error out"=w376:errorcluster, "Pixel Coordinates"=w387:cluster{"X":sgl, "Y":sgl})  [unwired: 3 in, 4 out]
      n254 = Bundle("Pixel Coordinates"=w388, "Pixel Coordinates"=w387, "Points for Arrow Overlay[2]"=w386, "Points for Arrow Overlay[3]"=w385) -> (w379:T5)  [unwired: 1 in]
      n255 = Merge Errors(w377, w376) -> (w375:errorcluster)
      n256 = Square(x=w416) -> (x^2=w419:dbl)
      n257 = Square(x=w420) -> (x^2=w418:dbl)
      n258 = Replace Array Subset(array=w380, new element=w379, index=w381) -> (w378:T1)
      n259 = Add(x=w419, y=w418) -> (x+y=w417:dbl)
      n260 = Square Root(x=w417) -> (sqrt(x)=w384:dbl)
      n261 = Replace Array Subset(array=w383, new element=w384, index=w381) -> (w382:dbl[])
    }
    frame "1853" {
      # "W1cos SVA -(W-W1)sin SVA"
      # "H'-W1 sin SVA"
      n262 = Search 1D Array(1D array=w471, element="H") -> (index of element=w439:i32)  [unwired: 1 in]
      n263 = Search 1D Array(1D array=w471, element="W") -> (index of element=w467:i32)  [unwired: 1 in]
      n264 = Search 1D Array(1D array=w471, element="W1") -> (index of element=w468:i32)  [unwired: 1 in]
      n265 = expression code="(x/180.0)*pi" "degrees to radians"(w463) -> (w480:dbl)
      n266 = Index Array(array=w438, index=w439) -> (element=w464:T4)
      n267 = Cosine(x=w480) -> (cos(x)=w479:dbl)
      n268 = Index Array(array=w441, index #1=w439, index #2=w468, index #3=w467) -> (element #1=w466:dbl, element #2=w465:dbl, element #3=w431:dbl)
      n269 = Sine(x=w480) -> (sin(x)=w430:dbl)
      n270 = Unbundle By Name(w464) -> ("Points for Arrow Overlay[0]"=w462:cluster{"X":sgl, "Y":sgl}, "Points for Arrow Overlay[1]"=w461:cluster{"X":sgl, "Y":sgl}, "Points for Arrow Overlay[2]"=w444:cluster{"X":sgl, "Y":sgl}, "Points for Arrow Overlay[3]"=w443:cluster{"X":sgl, "Y":sgl})
      n271 = Multiply(x=w465, y=w479) -> (x*y=w478:dbl)
      n272 = Multiply(x=w431, y=w430) -> (x*y=w428:dbl)
      n273 = Multiply(x=w465, y=w430) -> (x*y=w429:dbl)
      n274 = Subtract(x=w465, y=w431) -> (x-y=w427:dbl)
      n275 = Multiply(x=w427, y=w430) -> (x*y=w473:dbl)
      n276 = Subtract(x=w466, y=w429) -> (x-y=w474:dbl)
      n277 = call "IMAQ Convert Pixel to Real World"("error in (no error)"=w450, "Pixel Coordinates"=w462, "Calibrated Image"=w432) -> ("error out"=w449:errorcluster, "Real World Coordinates"=w460:cluster{"X":sgl, "Y":sgl})  [unwired: 3 in, 4 out]
      n278 = call "IMAQ Convert Pixel to Real World"("error in (no error)"=w450, "Pixel Coordinates"=w461, "Calibrated Image"=w432) -> ("error out"=w448:errorcluster, "Real World Coordinates"=w459:cluster{"X":sgl, "Y":sgl})  [unwired: 3 in, 4 out]
      n279 = Divide(x=w427, y=2.0) -> (x/y=w425:dbl)
      n280 = Subtract(x=w428, y=w425) -> ()  [unwired: 1 out]
      n281 = Unbundle By Name(w460) -> ("X"=w458:sgl, "Y"=w457:sgl)
      n282 = Subtract(x=w478, y=w473) -> (x-y=w424:dbl)
      n283 = Unbundle By Name(w459) -> ("X"=w453:sgl, "Y"=w455:sgl)
      n284 = Add(x=w424, y=w457) -> (x+y=w456:dbl)
      n285 = Add(x=w424, y=w455) -> (x+y=w454:dbl)
      n286 = Bundle("X"=w458, w456) -> (w452:cluster{"X":sgl, dbl})  [unwired: 1 in]
      n287 = Merge Errors(w449, w448) -> (w447:errorcluster)
      n288 = Bundle("X"=w453, w454) -> (w451:cluster{"X":sgl, dbl})  [unwired: 1 in]
      n289 = call "IMAQ Convert Real World to Pixel"("error in (no error)"=w447, "Real World Coordinates"=w452, "Calibrated Image"=w432) -> ("error out"=w435:errorcluster, "Pixel Coordinates"=w446:cluster{"X":sgl, "Y":sgl})  [unwired: 3 in, 4 out]
      n290 = call "IMAQ Convert Real World to Pixel"("error in (no error)"=w447, "Real World Coordinates"=w451, "Calibrated Image"=w432) -> ("error out"=w434:errorcluster, "Pixel Coordinates"=w445:cluster{"X":sgl, "Y":sgl})  [unwired: 3 in, 4 out]
      n291 = Bundle("Pixel Coordinates"=w446, "Pixel Coordinates"=w445, "Points for Arrow Overlay[2]"=w444, "Points for Arrow Overlay[3]"=w443) -> (w437:T5)  [unwired: 1 in]
      n292 = Merge Errors(w435, w434) -> (w433:errorcluster)
      n293 = Square(x=w474) -> (x^2=w477:dbl)
      n294 = Square(x=w424) -> (x^2=w476:dbl)
      n295 = Replace Array Subset(array=w438, new element=w437, index=w439) -> (w436:T1)
      n296 = Add(x=w477, y=w476) -> (x+y=w475:dbl)
      n297 = Square Root(x=w475) -> (sqrt(x)=w442:dbl)
      n298 = Replace Array Subset(array=w441, new element=w442, index=w439) -> (w440:dbl[])
    }
    frame "1525" {
      n299 = Search 1D Array(1D array=w491, element="W" ("y")) -> (index of element=w529:i32)  [unwired: 1 in]
      n300 = Subtract(x=90.0, y=w487) -> (x-y=w504:dbl)
      n301 = Search 1D Array(1D array=w491, element="H" ("y")) -> (index of element=w506:i32)  [unwired: 1 in]
      n302 = expression code="(x/180.0)*pi" "degrees to radians"(w504) -> (w524:dbl)
      n303 = expression code="(x/180.0)*pi" "degrees to radians"(w487) -> (w526:dbl)
      n304 = Index Array(array=w489, index=w529) -> (element=w528:dbl)
      n305 = Cosine(x=w524) -> (cos(x)=w523:dbl)
      n306 = Cosine(x=w526) -> (cos(x)=w525:dbl)
      n307 = Multiply(x=w528, y=w523) -> (x*y=w482:dbl)
      n308 = Multiply(x=w528, y=w525) -> (x*y=w503:dbl)
      n309 = Index Array(array=w489, index=w506) -> (element=w527:dbl)
      n310 = Index Array(array=w490, index=w506) -> (element=w518:T4)
      n311 = Unbundle By Name(w518) -> ("Points for Arrow Overlay[0]"=w517:cluster{"X":sgl, "Y":sgl}, "Points for Arrow Overlay[1]"=w516:cluster{"X":sgl, "Y":sgl}, "Points for Arrow Overlay[2]"=w509:cluster{"X":sgl, "Y":sgl}, "Points for Arrow Overlay[3]"=w508:cluster{"X":sgl, "Y":sgl})
      n312 = Subtract(x=w527, y=w482) -> (x-y=w481:dbl)
      n313 = Square(x=w481) -> (x^2=w521:dbl)
      n314 = Square(x=w503) -> (x^2=w522:dbl)
      n315 = call "IMAQ Convert Pixel to Real World"("error in (no error)"=w486, "Pixel Coordinates"=w517, "Calibrated Image"=w488) -> ("error out"=w494:errorcluster, "Real World Coordinates"=w496:cluster{"X":sgl, "Y":sgl})  [unwired: 3 in, 4 out]
      n316 = call "IMAQ Convert Pixel to Real World"("error in (no error)"=w486, "Pixel Coordinates"=w516, "Calibrated Image"=w488) -> ("error out"=w493:errorcluster, "Real World Coordinates"=w495:cluster{"X":sgl, "Y":sgl})  [unwired: 3 in, 4 out]
      n317 = Add(x=w522, y=w521) -> (x+y=w520:dbl)
      n318 = Unbundle By Name(w496) -> ("X"=w512:sgl, "Y"=w515:sgl)
      n319 = Unbundle By Name(w495) -> ("X"=w510:sgl, "Y"=w514:sgl)
      n320 = Add(x=w481, y=w515) -> (x+y=w513:dbl)
      n321 = Add(x=w481, y=w514) -> (x+y=w511:dbl)
      n322 = Square Root(x=w520) -> (sqrt(x)=w519:dbl)
      n323 = Bundle("X"=w512, w513) -> (w502:cluster{"X":sgl, dbl})  [unwired: 1 in]
      n324 = Merge Errors(w494, w493) -> (w492:errorcluster)
      n325 = Bundle("X"=w510, w511) -> (w500:cluster{"X":sgl, dbl})  [unwired: 1 in]
      n326 = Replace Array Subset(array=w489, new element=w519, index=w506) -> (w485:dbl[])
      n327 = call "IMAQ Convert Real World to Pixel"("error in (no error)"=w492, "Real World Coordinates"=w502, "Calibrated Image"=w488) -> ("error out"=w498:errorcluster, "Pixel Coordinates"=w501:cluster{"X":sgl, "Y":sgl})  [unwired: 3 in, 4 out]
      n328 = call "IMAQ Convert Real World to Pixel"("error in (no error)"=w492, "Real World Coordinates"=w500, "Calibrated Image"=w488) -> ("error out"=w497:errorcluster, "Pixel Coordinates"=w499:cluster{"X":sgl, "Y":sgl})  [unwired: 3 in, 4 out]
      n329 = Bundle("Pixel Coordinates"=w501, "Pixel Coordinates"=w499, "Points for Arrow Overlay[2]"=w509, "Points for Arrow Overlay[3]"=w508) -> (w507:T5)  [unwired: 1 in]
      n330 = Merge Errors(w498, w497) -> (w483:errorcluster)
      n331 = Replace Array Subset(array=w490, new element=w507, index=w506) -> (w484:T1)
    }
    frame "1524" {
      n332 = Search 1D Array(1D array=w542, element="W" ("y")) -> (index of element=w580:i32)  [unwired: 1 in]
      n333 = Subtract(x=90.0, y=w538) -> (x-y=w555:dbl)
      n334 = Search 1D Array(1D array=w542, element="H" ("y")) -> (index of element=w557:i32)  [unwired: 1 in]
      n335 = expression code="(x/180.0)*pi" "degrees to radians"(w555) -> (w575:dbl)
      n336 = expression code="(x/180.0)*pi" "degrees to radians"(w538) -> (w577:dbl)
      n337 = Index Array(array=w540, index=w580) -> (element=w579:dbl)
      n338 = Cosine(x=w575) -> (cos(x)=w574:dbl)
      n339 = Cosine(x=w577) -> (cos(x)=w576:dbl)
      n340 = Multiply(x=w579, y=w574) -> (x*y=w533:dbl)
      n341 = Multiply(x=w579, y=w576) -> (x*y=w554:dbl)
      n342 = Index Array(array=w540, index=w557) -> (element=w578:dbl)
      n343 = Index Array(array=w541, index=w557) -> (element=w569:T4)
      n344 = Unbundle By Name(w569) -> ("Points for Arrow Overlay[0]"=w568:cluster{"X":sgl, "Y":sgl}, "Points for Arrow Overlay[1]"=w567:cluster{"X":sgl, "Y":sgl}, "Points for Arrow Overlay[2]"=w560:cluster{"X":sgl, "Y":sgl}, "Points for Arrow Overlay[3]"=w559:cluster{"X":sgl, "Y":sgl})
      n345 = Subtract(x=w578, y=w533) -> (x-y=w532:dbl)
      n346 = Square(x=w532) -> (x^2=w572:dbl)
      n347 = Square(x=w554) -> (x^2=w573:dbl)
      n348 = call "IMAQ Convert Pixel to Real World"("error in (no error)"=w537, "Pixel Coordinates"=w568, "Calibrated Image"=w539) -> ("error out"=w545:errorcluster, "Real World Coordinates"=w547:cluster{"X":sgl, "Y":sgl})  [unwired: 3 in, 4 out]
      n349 = call "IMAQ Convert Pixel to Real World"("error in (no error)"=w537, "Pixel Coordinates"=w567, "Calibrated Image"=w539) -> ("error out"=w544:errorcluster, "Real World Coordinates"=w546:cluster{"X":sgl, "Y":sgl})  [unwired: 3 in, 4 out]
      n350 = Add(x=w573, y=w572) -> (x+y=w571:dbl)
      n351 = Unbundle By Name(w547) -> ("X"=w563:sgl, "Y"=w566:sgl)
      n352 = Unbundle By Name(w546) -> ("X"=w561:sgl, "Y"=w565:sgl)
      n353 = Add(x=w532, y=w566) -> (x+y=w564:dbl)
      n354 = Add(x=w532, y=w565) -> (x+y=w562:dbl)
      n355 = Square Root(x=w571) -> (sqrt(x)=w570:dbl)
      n356 = Bundle("X"=w563, w564) -> (w553:cluster{"X":sgl, dbl})  [unwired: 1 in]
      n357 = Merge Errors(w545, w544) -> (w543:errorcluster)
      n358 = Bundle("X"=w561, w562) -> (w551:cluster{"X":sgl, dbl})  [unwired: 1 in]
      n359 = Replace Array Subset(array=w540, new element=w570, index=w557) -> (w536:dbl[])
      n360 = call "IMAQ Convert Real World to Pixel"("error in (no error)"=w543, "Real World Coordinates"=w553, "Calibrated Image"=w539) -> ("error out"=w549:errorcluster, "Pixel Coordinates"=w552:cluster{"X":sgl, "Y":sgl})  [unwired: 3 in, 4 out]
      n361 = call "IMAQ Convert Real World to Pixel"("error in (no error)"=w543, "Real World Coordinates"=w551, "Calibrated Image"=w539) -> ("error out"=w548:errorcluster, "Pixel Coordinates"=w550:cluster{"X":sgl, "Y":sgl})  [unwired: 3 in, 4 out]
      n362 = Bundle("Pixel Coordinates"=w552, "Pixel Coordinates"=w550, "Points for Arrow Overlay[2]"=w560, "Points for Arrow Overlay[3]"=w559) -> (w558:T5)  [unwired: 1 in]
      n363 = Merge Errors(w549, w548) -> (w534:errorcluster)
      n364 = Replace Array Subset(array=w541, new element=w558, index=w557) -> (w535:T1)
    }
    frame "1891" {
      n365 = Search 1D Array(1D array=w593, element="W" ("y")) -> (index of element=w631:i32)  [unwired: 1 in]
      n366 = Subtract(x=90.0, y=w589) -> (x-y=w606:dbl)
      n367 = Search 1D Array(1D array=w593, element="H" ("y")) -> (index of element=w608:i32)  [unwired: 1 in]
      n368 = expression code="(x/180.0)*pi" "degrees to radians"(w606) -> (w626:dbl)
      n369 = expression code="(x/180.0)*pi" "degrees to radians"(w589) -> (w628:dbl)
      n370 = Index Array(array=w591, index=w631) -> (element=w630:dbl)
      n371 = Cosine(x=w626) -> (cos(x)=w625:dbl)
      n372 = Cosine(x=w628) -> (cos(x)=w627:dbl)
      n373 = Multiply(x=w630, y=w625) -> (x*y=w584:dbl)
      n374 = Multiply(x=w630, y=w627) -> (x*y=w605:dbl)
      n375 = Index Array(array=w591, index=w608) -> (element=w629:dbl)
      n376 = Index Array(array=w592, index=w608) -> (element=w620:T4)
      n377 = Unbundle By Name(w620) -> ("Points for Arrow Overlay[0]"=w619:cluster{"X":sgl, "Y":sgl}, "Points for Arrow Overlay[1]"=w618:cluster{"X":sgl, "Y":sgl}, "Points for Arrow Overlay[2]"=w611:cluster{"X":sgl, "Y":sgl}, "Points for Arrow Overlay[3]"=w610:cluster{"X":sgl, "Y":sgl})
      n378 = Subtract(x=w629, y=w584) -> (x-y=w583:dbl)
      n379 = Square(x=w583) -> (x^2=w623:dbl)
      n380 = Square(x=w605) -> (x^2=w624:dbl)
      n381 = call "IMAQ Convert Pixel to Real World"("error in (no error)"=w588, "Pixel Coordinates"=w619, "Calibrated Image"=w590) -> ("error out"=w596:errorcluster, "Real World Coordinates"=w598:cluster{"X":sgl, "Y":sgl})  [unwired: 3 in, 4 out]
      n382 = call "IMAQ Convert Pixel to Real World"("error in (no error)"=w588, "Pixel Coordinates"=w618, "Calibrated Image"=w590) -> ("error out"=w595:errorcluster, "Real World Coordinates"=w597:cluster{"X":sgl, "Y":sgl})  [unwired: 3 in, 4 out]
      n383 = Add(x=w624, y=w623) -> (x+y=w622:dbl)
      n384 = Unbundle By Name(w598) -> ("X"=w614:sgl, "Y"=w617:sgl)
      n385 = Unbundle By Name(w597) -> ("X"=w612:sgl, "Y"=w616:sgl)
      n386 = Add(x=w583, y=w617) -> (x+y=w615:dbl)
      n387 = Add(x=w583, y=w616) -> (x+y=w613:dbl)
      n388 = Square Root(x=w622) -> (sqrt(x)=w621:dbl)
      n389 = Bundle("X"=w614, w615) -> (w604:cluster{"X":sgl, dbl})  [unwired: 1 in]
      n390 = Merge Errors(w596, w595) -> (w594:errorcluster)
      n391 = Bundle("X"=w612, w613) -> (w602:cluster{"X":sgl, dbl})  [unwired: 1 in]
      n392 = Replace Array Subset(array=w591, new element=w621, index=w608) -> (w587:dbl[])
      n393 = call "IMAQ Convert Real World to Pixel"("error in (no error)"=w594, "Real World Coordinates"=w604, "Calibrated Image"=w590) -> ("error out"=w600:errorcluster, "Pixel Coordinates"=w603:cluster{"X":sgl, "Y":sgl})  [unwired: 3 in, 4 out]
      n394 = call "IMAQ Convert Real World to Pixel"("error in (no error)"=w594, "Real World Coordinates"=w602, "Calibrated Image"=w590) -> ("error out"=w599:errorcluster, "Pixel Coordinates"=w601:cluster{"X":sgl, "Y":sgl})  [unwired: 3 in, 4 out]
      n395 = Bundle("Pixel Coordinates"=w603, "Pixel Coordinates"=w601, "Points for Arrow Overlay[2]"=w611, "Points for Arrow Overlay[3]"=w610) -> (w609:T5)  [unwired: 1 in]
      n396 = Merge Errors(w600, w599) -> (w585:errorcluster)
      n397 = Replace Array Subset(array=w592, new element=w609, index=w608) -> (w586:T1)
    }
    frame "1892" {
      n398 = Subtract(x=90.0, y=w675) -> (x-y=w688:dbl)
      n399 = Search 1D Array(1D array=w669, element="H" ("y")) -> (index of element=w660:i32)  [unwired: 1 in]
      n400 = Search 1D Array(1D array=w669, element="W" ("y")) -> (index of element=w712:i32)  [unwired: 1 in]
      n401 = Search 1D Array(1D array=w669, element="H1" ("y")) -> (index of element=w634:i32)  [unwired: 1 in]
      n402 = expression code="(x/180.0)*pi" "degrees to radians"(w688) -> (w707:dbl)
      n403 = expression code="(x/180.0)*pi" "degrees to radians"(w675) -> (w709:dbl)
      n404 = Index Array(array=w676, index #1=w660, index #2=w634) -> (element #1=w710:dbl, element #2=w663:dbl)
      n405 = Index Array(array=w676, index=w712) -> (element=w711:dbl)
      n406 = Index Array(array=w677, index #1=w660, index #2=w634) -> (element #1=w701:T4, element #2=w668:T4)
      n407 = Cosine(x=w707) -> (cos(x)=w706:dbl)
      n408 = Unbundle By Name(w701) -> ("Points for Arrow Overlay[0]"=w700:cluster{"X":sgl, "Y":sgl}, "Points for Arrow Overlay[1]"=w699:cluster{"X":sgl, "Y":sgl}, "Points for Arrow Overlay[2]"=w692:cluster{"X":sgl, "Y":sgl}, "Points for Arrow Overlay[3]"=w691:cluster{"X":sgl, "Y":sgl})
      n409 = Unbundle By Name(w668) -> ("Points for Arrow Overlay[0]"=w656:cluster{"X":sgl, "Y":sgl}, "Points for Arrow Overlay[1]"=w655:cluster{"X":sgl, "Y":sgl}, "Points for Arrow Overlay[2]"=w659:cluster{"X":sgl, "Y":sgl}, "Points for Arrow Overlay[3]"=w658:cluster{"X":sgl, "Y":sgl})
      n410 = Multiply(x=w711, y=w706) -> (x*y=w662:dbl)
      n411 = Cosine(x=w709) -> (cos(x)=w708:dbl)
      n412 = Subtract(x=w710, y=w662) -> (x-y=w671:dbl)
      n413 = Subtract(x=w663, y=w662) -> (x-y=w649:dbl)
      n414 = Multiply(x=w711, y=w708) -> (x*y=w664:dbl)
      n415 = call "IMAQ Convert Pixel to Real World"("error in (no error)"=w657, "Pixel Coordinates"=w700, "Calibrated Image"=w643) -> ("error out"=w679:errorcluster, "Real World Coordinates"=w681:cluster{"X":sgl, "Y":sgl})  [unwired: 3 in, 4 out]
      n416 = call "IMAQ Convert Pixel to Real World"("error in (no error)"=w657, "Pixel Coordinates"=w699, "Calibrated Image"=w643) -> ("error out"=w678:errorcluster, "Real World Coordinates"=w680:cluster{"X":sgl, "Y":sgl})  [unwired: 3 in, 4 out]
      n417 = call "IMAQ Convert Pixel to Real World"("error in (no error)"=w657, "Pixel Coordinates"=w656, "Calibrated Image"=w643) -> ("error out"=w641:errorcluster, "Real World Coordinates"=w654:cluster{"X":sgl, "Y":sgl})  [unwired: 3 in, 4 out]
      n418 = call "IMAQ Convert Pixel to Real World"("error in (no error)"=w657, "Pixel Coordinates"=w655, "Calibrated Image"=w643) -> ("error out"=w642:errorcluster, "Real World Coordinates"=w653:cluster{"X":sgl, "Y":sgl})  [unwired: 3 in, 4 out]
      n419 = Square(x=w671) -> (x^2=w704:dbl)
      n420 = Square(x=w664) -> (x^2=w705:dbl)
      n421 = Square(x=w649) -> (x^2=w666:dbl)
      n422 = Square(x=w664) -> (x^2=w665:dbl)
      n423 = Unbundle By Name(w681) -> ("X"=w695:sgl, "Y"=w698:sgl)
      n424 = Unbundle By Name(w680) -> ("X"=w693:sgl, "Y"=w697:sgl)
      n425 = Unbundle By Name(w654) -> ("X"=w652:sgl, "Y"=w650:sgl)
      n426 = Unbundle By Name(w653) -> ("X"=w651:sgl, "Y"=w648:sgl)
      n427 = Add(x=w671, y=w698) -> (x+y=w696:dbl)
      n428 = Add(x=w671, y=w697) -> (x+y=w694:dbl)
      n429 = Add(x=w649, y=w650) -> (x+y=w647:dbl)
      n430 = Add(x=w649, y=w648) -> (x+y=w646:dbl)
      n431 = Add(x=w705, y=w704) -> (x+y=w703:dbl)
      n432 = Add(x=w665, y=w666) -> (x+y=w667:dbl)
      n433 = Bundle("X"=w695, w696) -> (w687:cluster{"X":sgl, dbl})  [unwired: 1 in]
      n434 = Merge Errors(w679, w678, w641, w642) -> (w637:errorcluster)
      n435 = Bundle("X"=w693, w694) -> (w685:cluster{"X":sgl, dbl})  [unwired: 1 in]
      n436 = Bundle("X"=w652, w647) -> (w644:cluster{"X":sgl, dbl})  [unwired: 1 in]
      n437 = Bundle("X"=w651, w646) -> (w645:cluster{"X":sgl, dbl})  [unwired: 1 in]
      n438 = Square Root(x=w703) -> (sqrt(x)=w702:dbl)
      n439 = Square Root(x=w667) -> (sqrt(x)=w661:dbl)
      n440 = call "IMAQ Convert Real World to Pixel"("error in (no error)"=w637, "Real World Coordinates"=w687, "Calibrated Image"=w643) -> ("error out"=w683:errorcluster, "Pixel Coordinates"=w686:cluster{"X":sgl, "Y":sgl})  [unwired: 3 in, 4 out]
      n441 = call "IMAQ Convert Real World to Pixel"("error in (no error)"=w637, "Real World Coordinates"=w685, "Calibrated Image"=w643) -> ("error out"=w682:errorcluster, "Pixel Coordinates"=w684:cluster{"X":sgl, "Y":sgl})  [unwired: 3 in, 4 out]
      n442 = call "IMAQ Convert Real World to Pixel"("error in (no error)"=w637, "Real World Coordinates"=w644, "Calibrated Image"=w643) -> ("error out"=w636:errorcluster, "Pixel Coordinates"=w639:cluster{"X":sgl, "Y":sgl})  [unwired: 3 in, 4 out]
      n443 = call "IMAQ Convert Real World to Pixel"("error in (no error)"=w637, "Real World Coordinates"=w645, "Calibrated Image"=w643) -> ("error out"=w635:errorcluster, "Pixel Coordinates"=w640:cluster{"X":sgl, "Y":sgl})  [unwired: 3 in, 4 out]
      n444 = Replace Array Subset(array=w676, new element #1=w702, index #1=w660, new element #2=w661, index #2=w634) -> (w674:dbl[])
      n445 = Bundle("Pixel Coordinates"=w686, "Pixel Coordinates"=w684, "Points for Arrow Overlay[2]"=w692, "Points for Arrow Overlay[3]"=w691) -> (w690:T5)  [unwired: 1 in]
      n446 = Bundle("Pixel Coordinates"=w639, "Pixel Coordinates"=w640, "Points for Arrow Overlay[2]"=w659, "Points for Arrow Overlay[3]"=w658) -> (w638:T5)  [unwired: 1 in]
      n447 = Merge Errors(w683, w682, w636, w635) -> (w672:errorcluster)
      n448 = Replace Array Subset(array=w677, new element #1=w690, index #1=w660, new element #2=w638, index #2=w634) -> (w673:T1)
    }
    frame "1828" {
      n449 = Search 1D Array(1D array=w725, element="W" ("y")) -> (index of element=w763:i32)  [unwired: 1 in]
      n450 = Subtract(x=90.0, y=w721) -> (x-y=w738:dbl)
      n451 = expression code="(x/180.0)*pi" "degrees to radians"(w738) -> (w758:dbl)
      n452 = expression code="(x/180.0)*pi" "degrees to radians"(w721) -> (w760:dbl)
      n453 = Search 1D Array(1D array=w725, element="H1" ("y")) -> (index of element=w740:i32)  [unwired: 1 in]
      n454 = Index Array(array=w723, index=w763) -> (element=w762:dbl)
      n455 = Cosine(x=w758) -> (cos(x)=w757:dbl)
      n456 = Cosine(x=w760) -> (cos(x)=w759:dbl)
      n457 = Multiply(x=w762, y=w757) -> (x*y=w716:dbl)
      n458 = Multiply(x=w762, y=w759) -> (x*y=w737:dbl)
      n459 = Index Array(array=w723, index=w740) -> (element=w761:dbl)
      n460 = Index Array(array=w724, index=w740) -> (element=w752:T4)
      n461 = Unbundle By Name(w752) -> ("Points for Arrow Overlay[0]"=w751:cluster{"X":sgl, "Y":sgl}, "Points for Arrow Overlay[1]"=w750:cluster{"X":sgl, "Y":sgl}, "Points for Arrow Overlay[2]"=w743:cluster{"X":sgl, "Y":sgl}, "Points for Arrow Overlay[3]"=w742:cluster{"X":sgl, "Y":sgl})
      n462 = Subtract(x=w761, y=w716) -> (x-y=w715:dbl)
      n463 = Square(x=w715) -> (x^2=w755:dbl)
      n464 = Square(x=w737) -> (x^2=w756:dbl)
      n465 = call "IMAQ Convert Pixel to Real World"("error in (no error)"=w720, "Pixel Coordinates"=w751, "Calibrated Image"=w722) -> ("error out"=w728:errorcluster, "Real World Coordinates"=w730:cluster{"X":sgl, "Y":sgl})  [unwired: 3 in, 4 out]
      n466 = call "IMAQ Convert Pixel to Real World"("error in (no error)"=w720, "Pixel Coordinates"=w750, "Calibrated Image"=w722) -> ("error out"=w727:errorcluster, "Real World Coordinates"=w729:cluster{"X":sgl, "Y":sgl})  [unwired: 3 in, 4 out]
      n467 = Add(x=w756, y=w755) -> (x+y=w754:dbl)
      n468 = Unbundle By Name(w730) -> ("X"=w746:sgl, "Y"=w749:sgl)
      n469 = Unbundle By Name(w729) -> ("X"=w744:sgl, "Y"=w748:sgl)
      n470 = Add(x=w715, y=w749) -> (x+y=w747:dbl)
      n471 = Add(x=w715, y=w748) -> (x+y=w745:dbl)
      n472 = Square Root(x=w754) -> (sqrt(x)=w753:dbl)
      n473 = Bundle("X"=w746, w747) -> (w736:cluster{"X":sgl, dbl})  [unwired: 1 in]
      n474 = Merge Errors(w728, w727) -> (w726:errorcluster)
      n475 = Bundle("X"=w744, w745) -> (w734:cluster{"X":sgl, dbl})  [unwired: 1 in]
      n476 = Replace Array Subset(array=w723, new element=w753, index=w740) -> (w719:dbl[])
      n477 = call "IMAQ Convert Real World to Pixel"("error in (no error)"=w726, "Real World Coordinates"=w736, "Calibrated Image"=w722) -> ("error out"=w732:errorcluster, "Pixel Coordinates"=w735:cluster{"X":sgl, "Y":sgl})  [unwired: 3 in, 4 out]
      n478 = call "IMAQ Convert Real World to Pixel"("error in (no error)"=w726, "Real World Coordinates"=w734, "Calibrated Image"=w722) -> ("error out"=w731:errorcluster, "Pixel Coordinates"=w733:cluster{"X":sgl, "Y":sgl})  [unwired: 3 in, 4 out]
      n479 = Bundle("Pixel Coordinates"=w735, "Pixel Coordinates"=w733, "Points for Arrow Overlay[2]"=w743, "Points for Arrow Overlay[3]"=w742) -> (w741:T5)  [unwired: 1 in]
      n480 = Merge Errors(w732, w731) -> (w717:errorcluster)
      n481 = Replace Array Subset(array=w724, new element=w741, index=w740) -> (w718:T1)
    }
  }
  "Measurement Results" <- w6
  "Points for Array Overlay Out" <- w3
  "error IO" <- w1
